vi "Visible or Invisible.vi"(9 "Visible":bool, 11 "Ctl Refnum":refnum<vi>) -> (3 "Ctl Refnum Out":refnum<vi>)   [LabVIEW 2024]
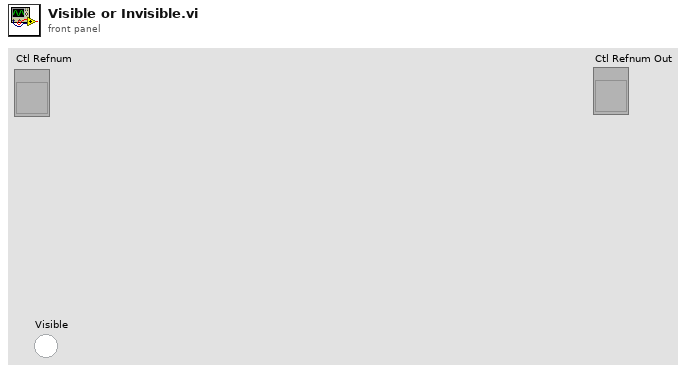
[diagram p1: front panel]
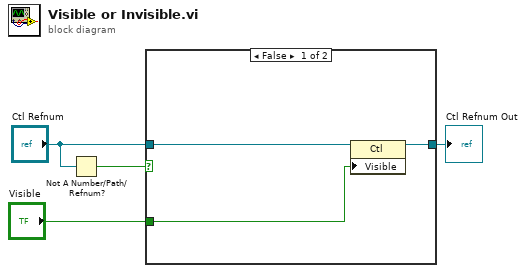
[diagram p0: block diagram]
diagram:
  n1 = Not A Number/Path/Refnum?(number/path/refnum="Ctl Refnum") -> (NaN/Path/Refnum?=w3:bool)
  n2 = case shown="False" w3 {
    tunnel: "Ctl Refnum" -> [w7 w8]
    tunnel: [w6 w8] -> w2
    tunnel: "Visible" -> [w5 _]
    frame False {
      n3 = property class="Ctl"(reference=w7, "Visible"=w5) -> (reference out=w6:refnum<vi>)  [unwired: 1 in, 1 out]
    }
    frame True {
    }
  }
  "Ctl Refnum Out" <- w2
